vi "Common.vi"(9 "Action":T1=enum."TemplatesFolderName") -> (1 "Output":string)   [LabVIEW 2016, in "NIVS_Consolidated_CDW_MetaDataObj.lvclass"]
doc: "Contains all constants, which are not part of specific part of the wizard."
uses:
  NIVS_Consolidated_CDW_MetaDataObj.lvclass
  Common.ctl
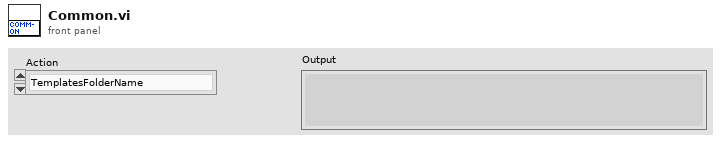
[diagram p1: front panel]
types:
  T1 = typedef "NIVS_Consolidated_CDW_MetaDataObj.lvclass/Common.ctl" = enum16{"ProjectName", "TemplatesFolderName", "ProjectTemplatePathAndName", "TimingAndSyncFolderName", "CustomDeviceFolderName", "PathToTemplates", "PathToConfigurationFile", "ProjectConfigurationName"}
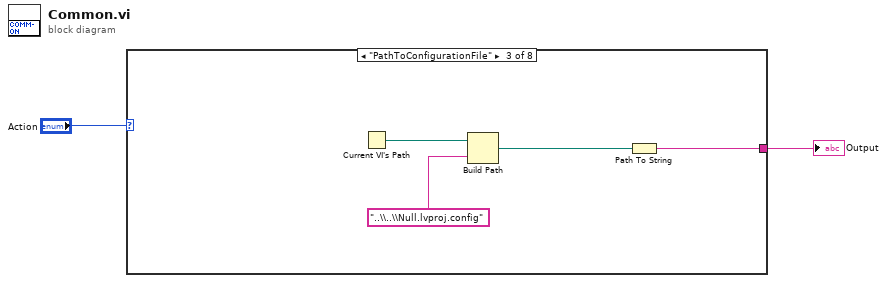
[diagram p0: block diagram]
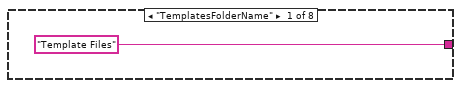
[diagram p2: hidden frame]
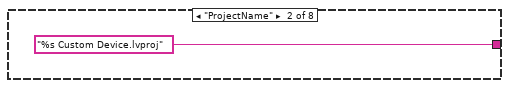
[diagram p3: hidden frame]
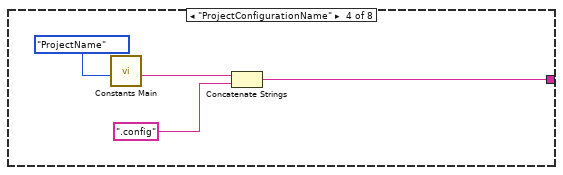
[diagram p4: hidden frame]
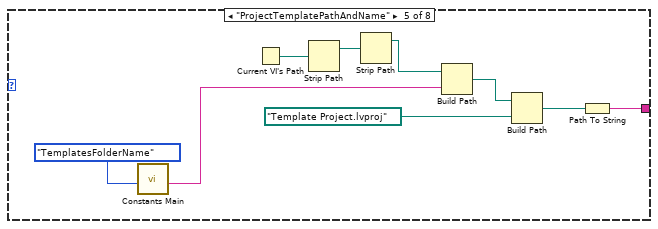
[diagram p5: hidden frame]
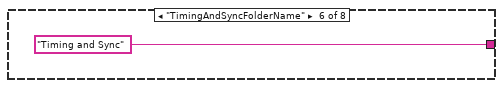
[diagram p6: hidden frame]
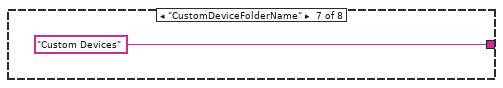
[diagram p7: hidden frame]
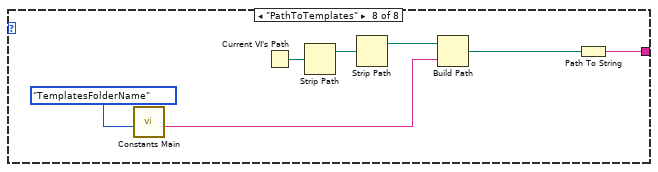
[diagram p8: hidden frame]
diagram:
  n1 = case shown="\"PathToConfigurationFile\"" "Action" {
    tunnel: ["Template Files" "%s Custom Device.lvproj" w8 w9 w16 "Timing and Sync" "Custom Devices" w24] -> w2
    frame "TemplatesFolderName" {
    }
    frame "ProjectName" {
    }
    frame "PathToConfigurationFile" {
      n2 = Current VI's Path() -> (path=w5:path)
      n3 = Build Path(base path=w5, name or relative path="..\\..\\Null.lvproj.config") -> (appended path=w6:path)
      n4 = Path To String(path=w6) -> (string=w8:string)
    }
    frame "ProjectConfigurationName" {
      n5 = call-poly "Constants Main.vi"("Action"=Common."ProjectName") -> ("Output"=w11:string)  [unwired: 10 in]
      n6 = Concatenate Strings(w11, ".config") -> (w9:string)
    }
    frame "ProjectTemplatePathAndName" {
      n7 = call-poly "Constants Main.vi"("Action"=Common."TemplatesFolderName") -> ("Output"=w21:string)  [unwired: 10 in]
      n8 = Current VI's Path() -> (path=w15:path)
      n9 = Strip Path(path=w15) -> (stripped path=w14:path)  [unwired: 1 out]
      n10 = Strip Path(path=w14) -> (stripped path=w13:path)  [unwired: 1 out]
      n11 = Build Path(base path=w13, name or relative path=w21) -> (appended path=w20:path)
      n12 = Build Path(base path=w20, name or relative path=path "Template Project.lvproj") -> (appended path=w18:path)
      n13 = Path To String(path=w18) -> (string=w16:string)
    }
    frame "TimingAndSyncFolderName" {
    }
    frame "CustomDeviceFolderName" {
    }
    frame "PathToTemplates" {
      n14 = call-poly "Constants Main.vi"("Action"=Common."TemplatesFolderName") -> ("Output"=w30:string)  [unwired: 10 in]
      n15 = Current VI's Path() -> (path=w27:path)
      n16 = Strip Path(path=w27) -> (stripped path=w26:path)  [unwired: 1 out]
      n17 = Strip Path(path=w26) -> (stripped path=w25:path)  [unwired: 1 out]
      n18 = Build Path(base path=w25, name or relative path=w30) -> (appended path=w29:path)
      n19 = Path To String(path=w29) -> (string=w24:string)
    }
  }
  "Output" <- w2
